vi "Solver_002.vi"(10 "Word List":string[](array[string])=["YELLOW", "ORANGE", "PURPLE", "BLUE", "GREEN", "RED"], 11 "Word Search Grid":string[][](array[string])=[["R", "B", "L", "U", "E", "W"], ["E", "G", "N", "A", "R", "O"], ["D", "B", "C", "E", "W", "L"], ["L", "L", "D", "K", "V", "L"], ["P", "U", "R", "P", "L", "E"], ["N", "E", "E", "R", "G", "Y"]]) -> (3 "Solutions":T1={"BLUE"=[{"Row"=0, "Column"=1}, {"Row"=0, "Column"=2}, {"Row"=0, "Column"=3}, {"Row"=0, "Column"=4}], "GREEN"=[{"Row"=5, "Column"=4}, {"Row"=5, "Column"=3}, {"Row"=5, "Column"=2}, {"Row"=5, "Column"=1}, {"Row"=5, "Column"=0}], "ORANGE"=[{"Row"=1, "Column"=5}, {"Row"=1, "Column"=4}, {"Row"=1, "Column"=3}, {"Row"=1, "Column"=2}, {"Row"=1, "Column"=1}, {"Row"=1, "Column"=0}], "PURPLE"=[{"Row"=4, "Column"=0}, {"Row"=4, "Column"=1}, {"Row"=4, "Column"=2}, {"Row"=4, "Column"=3}, {"Row"=4, "Column"=4}, {"Row"=4, "Column"=5}], "RED"=[{"Row"=0, "Column"=0}, {"Row"=1, "Column"=0}, {"Row"=2, "Column"=0}], "YELLOW"=[{"Row"=5, "Column"=5}, {"Row"=4, "Column"=5}, {"Row"=3, "Column"=5}, {"Row"=2, "Column"=5}, {"Row"=1, "Column"=5}, {"Row"=0, "Column"=5}]})   [LabVIEW 2022 SP3]
uses:
  Solutions--map.ctl
  Letter Index--cluster.ctl
panel:
  # "Do not change the connector pane of this VI."
  # "Observe the default values stored in this VI to understand how each word is represented in the Solutions map.\n\nSee the block diagram for a simple implementation of a solution. Note that this approach is not very efficient, and you will want to come up with a faster way to find the words in the grid."
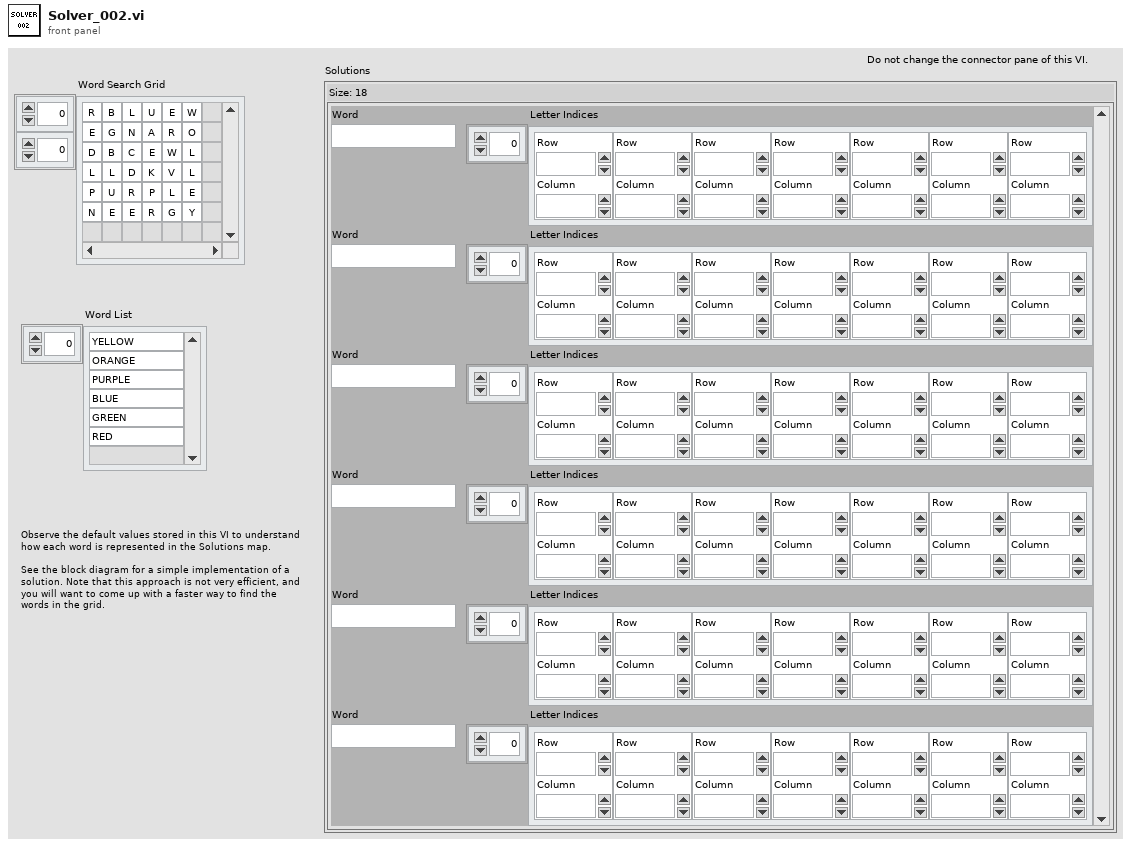
[diagram p1: front panel]
types:
  T1 = typedef "Solutions--map.ctl" = map{string, T2[]}
  T2 = typedef "Letter Index--cluster.ctl" = cluster{"Row":i32, "Column":i32}
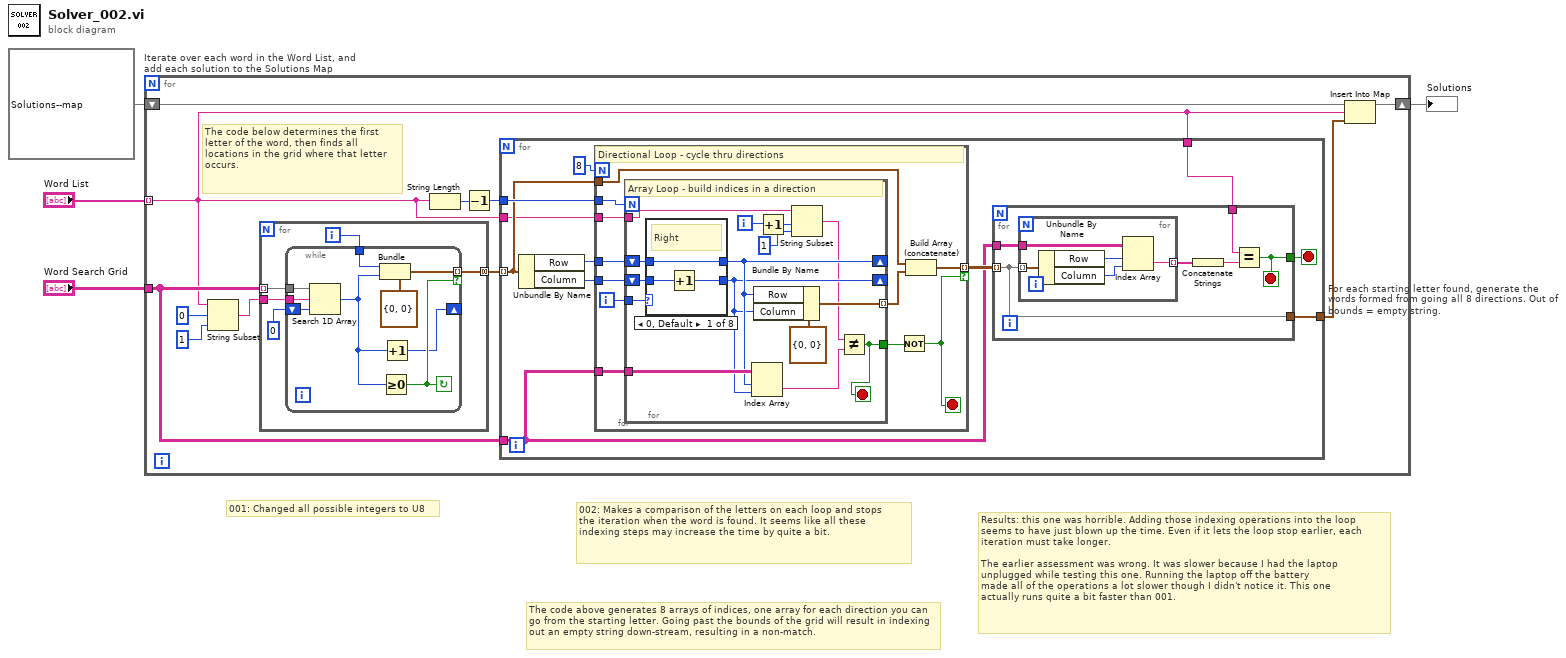
[diagram p0: block diagram]
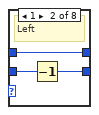
[diagram p2: hidden frame]
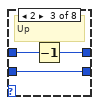
[diagram p3: hidden frame]
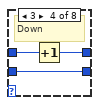
[diagram p4: hidden frame]
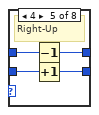
[diagram p5: hidden frame]
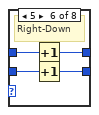
[diagram p6: hidden frame]
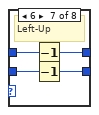
[diagram p7: hidden frame]
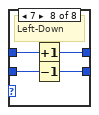
[diagram p8: hidden frame]
diagram:
  # "Results: this one was horrible. Adding those indexing operations into the loop\nseems to have just blown up the time. Even if it lets the loop stop earlier, each\niteration must take longer.\n\nThe earlier assessment was wrong. It was slower because I had the laptop \nunplugged while testing this one. Running the laptop off the battery \nmade all of the operations a lot slower though I didn't notice it. This one \nactually runs quite a bit faster than 001."
  # "002: Makes a comparison of the letters on each loop and stops \nthe iteration when the word is found. It seems like all these \nindexing steps may increase the time by quite a bit."
  # "001: Changed all possible integers to U8"
  # "The code above generates 8 arrays of indices, one array for each direction you can go from the starting letter. Going past the bounds of the grid will result in indexing out an empty string down-stream, resulting in a non-match."
  n1 = for "Iterate over each word in the Word List, and add each solution to the Solutions Map" {
    tunnel: "Word Search Grid" -> [w7]
    tunnel: "Word List" -> [w5] mode=indexing
    shift-right: [w14] -> w4
    shift-left: T1 {} ("Solutions") -> [w15]
    # "The code below determines the first letter of the word, then finds all locations in the grid where that letter occurs."
    n2 = String Subset(string=w5, offset (0)=u8 0, length (rest)=u8 1 ("length (rest)")) -> (substring=w12:string)
    n3 = for {
      tunnel: w7 -> [w96] mode=indexing
      tunnel: w12 -> [w95]
      tunnel: [w93] -> w11 mode=concatenating
      i -> [w94]
      n4 = while {
        tunnel: w96 -> [w105]
        tunnel: w95 -> [w104]
        tunnel: w94 -> [w102]
        tunnel: [w101] -> w93 mode=indexing if=w100
        shift-right: [w97] -> _
        shift-left: 0 -> [w99]
        stop <- w100 continue-if-true
        n5 = Search 1D Array(1D array=w105, element=w104, start index (0)=w99) -> (index of element=w98:i32)
        n6 = Bundle(cluster=T2 {"Row"=0, "Column"=0} ("Letter Index"), "Row"=w102, "Column"=w98) -> (w101:T2)
        n7 = Greater Or Equal To 0?(x=w98) -> (x >= 0?=w100:bool)
        n8 = Increment(x=w98) -> (x+1=w97:i32)
      }
    }
    n9 = String Length(string=w5) -> (length=w9:i32)
    n10 = Decrement(x=w9) -> (x-1=w8:i32)
    n11 = for "For each starting letter found, generate the words formed from going all 8 directions. Out of bounds = empty string." {
      tunnel: w11 -> [w22] mode=indexing
      tunnel: w8 -> [w25]
      tunnel: w7 -> [w16]
      tunnel: [w20] -> w6
      tunnel: w5 -> [w19]
      tunnel: w5 -> [w17]
      stop <- w18 stop-if-true
      n12 = Unbundle By Name(w22) -> ("Row"=w24:i32, "Column"=w23:i32)
      n13 = for {
        N: 8 -> [_]
        tunnel: w25 -> [w48]
        tunnel: w24 -> [w47]
        tunnel: w23 -> [w46]
        tunnel: w22 -> [w43]
        tunnel: [w42] -> w21 mode=indexing if=w38
        tunnel: w17 -> [w41]
        tunnel: w16 -> [w40]
        i -> [w45]
        stop <- w38 stop-if-true
        # "Directional Loop - cycle thru directions"
        n14 = for {
          N: w48 -> [_]
          tunnel: w45 -> [w61]
          tunnel: [w59] -> w44 mode=indexing
          shift-right: [w55] -> _
          shift-left: w47 -> [w63]
          shift-right: [w54] -> _
          shift-left: w46 -> [w62]
          tunnel: [w49] -> w39
          tunnel: w41 -> [w57]
          tunnel: w40 -> [w56]
          i -> [w53]
          stop <- w49 stop-if-true
          # "Array Loop - build indices in a direction"
          n15 = case shown="0, Default" w61 {
            tunnel: w63 -> [w64 w67 w71 w74 w78 w82 w86 w90]
            tunnel: w62 -> [w66 w69 w72 w75 w79 w83 w87 w91]
            tunnel: [w65 w68 w72 w75 w76 w80 w84 w88] -> w54
            tunnel: [w64 w67 w70 w73 w77 w81 w85 w89] -> w55
            frame 0, Default {
              # "Right"
              n16 = Increment(x=w66) -> (x+1=w65:i32)
            }
            frame 1 {
              # "Left"
              n17 = Decrement(x=w69) -> (x-1=w68:i32)
            }
            frame 2 {
              # "Up"
              n18 = Decrement(x=w71) -> (x-1=w70:i32)
            }
            frame 3 {
              # "Down"
              n19 = Increment(x=w74) -> (x+1=w73:i32)
            }
            frame 4 {
              # "Right-Up"
              n20 = Decrement(x=w78) -> (x-1=w77:i32)
              n21 = Increment(x=w79) -> (x+1=w76:i32)
            }
            frame 5 {
              # "Right-Down"
              n22 = Increment(x=w82) -> (x+1=w81:i32)
              n23 = Increment(x=w83) -> (x+1=w80:i32)
            }
            frame 6 {
              # "Left-Up"
              n24 = Decrement(x=w86) -> (x-1=w85:i32)
              n25 = Decrement(x=w87) -> (x-1=w84:i32)
            }
            frame 7 {
              # "Left-Down"
              n26 = Increment(x=w90) -> (x+1=w89:i32)
              n27 = Decrement(x=w91) -> (x-1=w88:i32)
            }
          }
          n28 = Index Array(array=w56, index (row)=w55, index (col)=w54) -> (element=w51:string)
          n29 = Bundle By Name(cluster=T2 {"Row"=0, "Column"=0} ("Letter Index"), "Row"=w55, "Column"=w54) -> (w59:T2)
          n30 = Increment(x=w53) -> (x+1=w52:i32)
          n31 = String Subset(string=w57, offset (0)=w52, length (rest)=1 ("length (rest)")) -> (substring=w50:string)
          n32 = Not Equal?(x=w50, y=w51) -> (x != y?=w49:bool)
        }
        n33 = Not(x=w39) -> (.not. x?=w38:bool)
        n34 = Build Array (concatenate)(w43, w44) -> (w42:T2[])
      }
      n35 = for {
        tunnel: w21 -> [w29] mode=indexing
        tunnel: w16 -> [w32]
        tunnel: [w29] -> w20
        tunnel: w19 -> [w28]
        tunnel: [w27] -> w18
        stop <- w27 stop-if-true
        n36 = for {
          tunnel: w29 -> [w37] mode=indexing
          tunnel: w32 -> [w35]
          tunnel: [w33] -> w31 mode=indexing
          n37 = Unbundle By Name(w37) -> ("Row"=w36:i32, "Column"=w34:i32)
          n38 = Index Array(array=w35, index (row)=w36, index (col)=w34) -> (element=w33:string)
        }
        n39 = Concatenate Strings(w31) -> (w30:string)
        n40 = Equal?(x=w28, y=w30) -> (x = y?=w27:bool)
      }
    }
    n41 = Insert Into Map(map in=w15, key=w5, value=w6) -> (map out=w14:T1)  [unwired: 2 out]
  }
  "Solutions" <- w4
